vi "Get Cell (String).vi"(8 "error in (no error)":errorcluster, 9 "Column":i32, 10 "Row":i32, 11 "Excel Legacy in":refnum<class "Excel Legacy.lvclass">) -> (0 "error out":errorcluster, 3 "Excel Legacy out":refnum<class "Excel Legacy.lvclass">, 5 "Value":string)   [LabVIEW 2013, in "Excel Legacy.lvclass"]
uses:
  Excel Legacy.lvclass
  Spreadsheet.lvclass
  Excel Legacy.lvclass/Excel Legacy.ctl
  C:/PhaeronGit/LVNPOI/Resources/NPOI 2.1.1 dotnet2/NPOI.dll
  Resources/NPOI 2.1.1 dotnet2/NPOI.dll
  <vilib>/ErrorRing/Error Ring.xnode
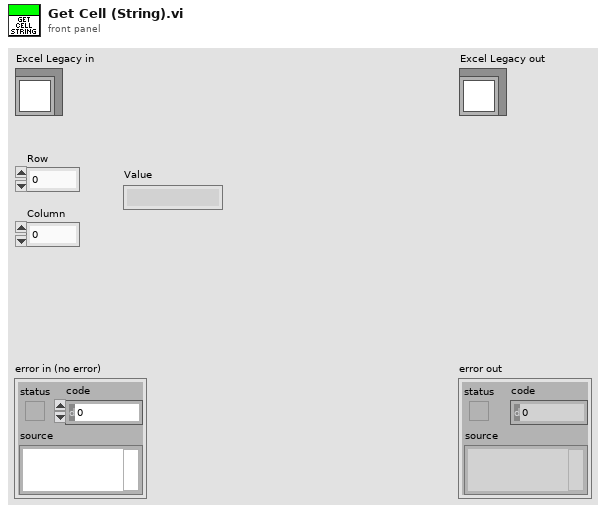
[diagram p1: front panel]
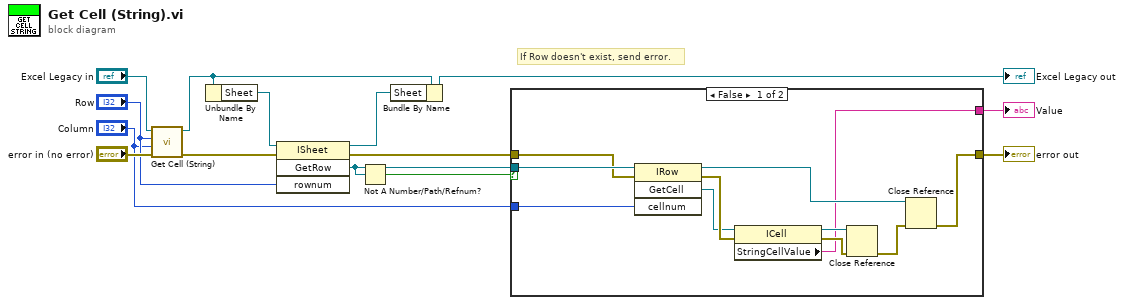
[diagram p0: block diagram]
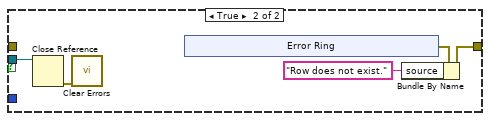
[diagram p2: hidden frame]
diagram:
  # "If Row doesn't exist, send error."
  n1 = call-parent "Get Cell (String).vi"("error in (no error)"="error in (no error)", "Column"="Column", "Row"="Row", "Spreadsheet in"="Excel Legacy in") -> ("error out"=w9:errorcluster, "Spreadsheet out"=w4:refnum<class "Excel Legacy.lvclass">)  [unwired: 5 in, 1 out]
  n2 = Unbundle By Name(w4) -> ("Sheet"=w3:refnum<k24>)
  n3 = invoke class="ISheet" method="GetRow"(reference=w3, error in=w9, "rownum"="Row") -> (reference out=w1:refnum<k24>, error out=w11:errorcluster, "GetRow"=w10:refnum<k24>)  [unwired: 1 in, 1 out]
  n4 = Not A Number/Path/Refnum?(number/path/refnum=w10) -> (NaN/Path/Refnum?=w12:bool)
  n5 = Bundle By Name(cluster=w4, "Sheet"=w1) -> (→"Excel Legacy out":refnum<class "Excel Legacy.lvclass">)
  n6 = case shown="False" w12 {
    tunnel: "Column" -> [w24 _]
    tunnel: [w22 w27] -> w6
    tunnel: w10 -> [w21 w30]
    tunnel: w11 -> [w20 _]
    tunnel: [w15 _] -> w5
    frame False {
      n7 = invoke class="IRow" method="GetCell"(reference=w21, error in=w20, "cellnum"=w24) -> (reference out=w25:refnum<k24>, error out=w19:errorcluster, "GetCell"=w18:refnum<k24>)  [unwired: 1 in, 1 out]
      n8 = property class="ICell"(reference=w18, error in=w19) -> (reference out=w16:refnum<k24>, error out=w17:errorcluster, "StringCellValue"=w15:string)
      n9 = Close Reference(reference=w16, error in (no error)=w17) -> (error out=w23:errorcluster)
      n10 = Close Reference(reference=w25, error in (no error)=w23) -> (error out=w22:errorcluster)
    }
    frame True {
      n11 = Close Reference(reference=w30) -> (error out=w29:errorcluster)  [unwired: 1 in]
      n12 = call <vilib>:"Clear Errors.vi"("error in (no error)"=w29) -> ()  [unwired: 6 in, 1 out]
      n13 = xnode "Error Ring"() -> ("error out"=w28:errorcluster)
      n14 = Bundle By Name(cluster=w28, "source"="Row does not exist.") -> (w27:errorcluster)
    }
  }
  "error out" <- w6
  "Value" <- w5
